vi "AssertRefnum.vi"(7 "Message (\"\")":string, 8 "error in (no error)":errorcluster, 10 "Refnum":variant) -> (0 "error out":errorcluster)   [LabVIEW 2017, in "Assertion.lvlib"]
doc: "Asserts that a variable is a valid refnum. Does nothing if an error occurred before this node runs. Returns an error if the assertion failed. Optionally adds a message to the error message if the assertion failed."
uses:
  Assertion.lvlib
  Constraint/IsRefnum/IsRefnum.lvclass
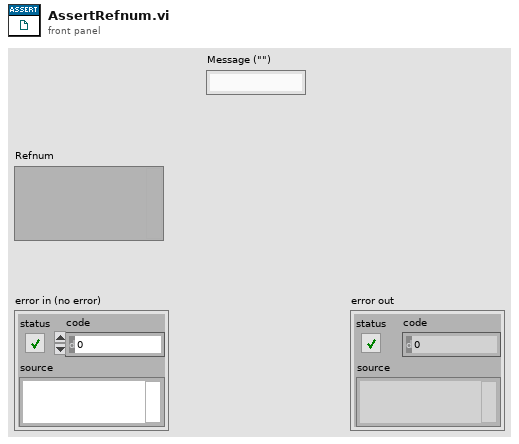
[diagram p1: front panel]
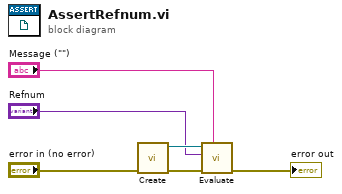
[diagram p0: block diagram]
diagram:
  n1 = call "Create.vi"("error in (no error)"="error in (no error)") -> ("error out"=w5:errorcluster, "IsRefnum"=w4:refnum<class "IsRefnum.lvclass">)  [unwired: 9 in]
  n2 = call-dynamic "Evaluate.vi"("Message (\"\")"="Message (\"\")", "error in (no error)"=w5, "Actual"="Refnum", "Constraint in"=w4) -> ("error out"=→"error out":errorcluster)  [unwired: 6 in, 1 out]
